vi "fgv_vlp16_config.vi"(7 "cmd":enum16{"read", "write"}(ring)=enum."write", 11 "VLP16 cfg":T1={"h range"={0, -85}, "v range"={0, -8}, "bounding box arr"=[]} {"v range" scale=-15.0..15.0; "h range" scale=-180.0..180.0}) -> (3 "VLP16 cfg out":T1={"h range"={0, -85}, "v range"={0, -8}, "bounding box arr"=[]} {"v range" scale=-15.0..15.0; "h range" scale=-180.0..180.0})   [LabVIEW 2019]
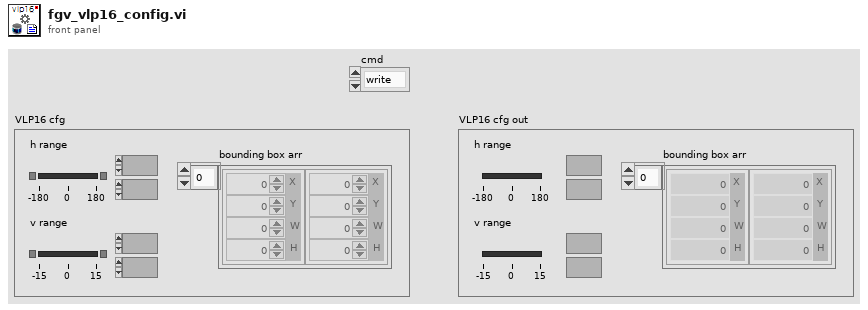
[diagram p1: front panel]
types:
  T1 = cluster{"h range":cluster{i16, i16}, "v range":cluster{i8, i8}, "bounding box arr":cluster{"X":dbl, "Y":dbl, "W":dbl, "H":dbl}[]}
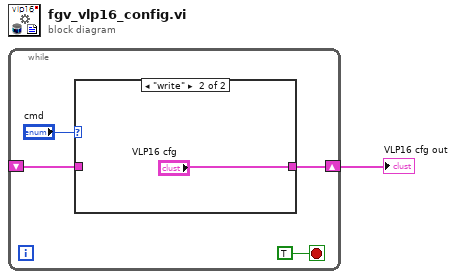
[diagram p0: block diagram]
diagram:
  n1 = while {
    shift-right: [w3] -> w1
    shift-left: _ -> [w2]
    stop <- TRUE stop-if-true
    n2 = case shown="\"write\"" "cmd" {
      tunnel: [w6 "VLP16 cfg"] -> w3
      tunnel: w2 -> [w6 _]
      frame "read", Default {
      }
      frame "write" {
      }
    }
  }
  "VLP16 cfg out" <- w1
